vi "Channel Page.vi"(8 "error in (no error)":errorcluster, 11 "Node Ptr":T3 format="%.0x") -> (0 "error out":errorcluster)   [LabVIEW 2011, in "IVI DC Power Supply Custom Device.lvlib"]
uses:
  IVI DC Power Supply Custom Device.lvlib
  <vilib>/NI Veristand/Custom Device API/Custom Device Item Ref.ctl
  current behaviour.ctl
  Global.vi
  <vilib>/NI Veristand/Custom Device Tools/Custom Device Utility Library/NI VeriStand - Search for All Items by GUID.vi
  <vilib>/NI Veristand/Custom Device API/Get Item Property (U16).vi
  <vilib>/NI Veristand/Custom Device API/Get Item Property (Double).vi
  <vilib>/NI Veristand/Custom Device API/Get Item Property (Boolean).vi
  <vilib>/NI Veristand/Custom Device API/Set Item Property (U16).vi
  <vilib>/NI Veristand/Custom Device API/Set Item Property (Double).vi
  <vilib>/NI Veristand/Custom Device Tools/Custom Device Utility Library/NI VeriStand - Search for Item by Name.vi
  <vilib>/NI Veristand/Custom Device API/Set Item Property (Boolean).vi
  <vilib>/NI Veristand/Custom Device API/Custom Device API.lvlib
  <vilib>/NI Veristand/Custom Device Tools/Custom Device Utility Library/Custom Device Utility Library.lvlib
panel:
  in  "Limit Behaviour":T1
  in  "OVP Limt (0.0 Volts)":dbl
  in  "OPV enabled":bool
  in  "Current Limit":dbl
  in  "Output Voltage":dbl
  in  "Channel #":T2(ring)
  in  "Header":cluster{"Section Name":string}={"Section Name"="IVI DC Power Supply Channel Settings"}
  in  "Description":string
  in  "Name":string
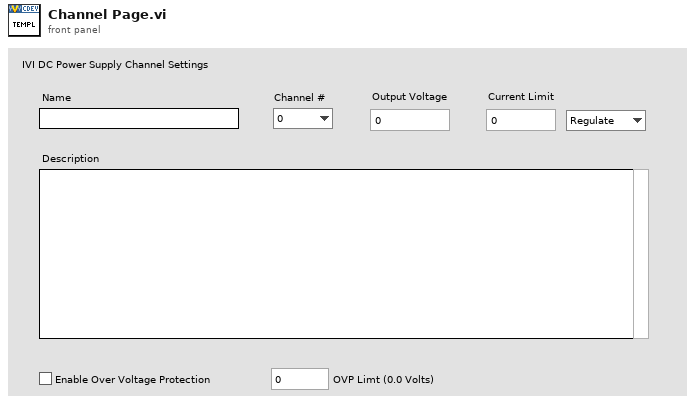
[diagram p1: front panel]
types:
  T1 = typedef "IVI DC Power Supply Custom Device.lvlib/current behaviour.ctl" = enum16{"Regulate", "Trip"}
  T2 = enum16{"0", "1", "2", "3", "4", "5", "6", "7", "8"}
  T3 = typedef "Custom Device API.lvlib/Custom Device Item Ref.ctl" = u64
  T4 = typedef "Custom Device API.lvlib/Custom Device Item Info.ctl" = cluster{"Name":string, "Is Channel":bool, "GUID":string}
  T5 = typedef "Custom Device API.lvlib/Custom Device Commands.ctl" = enum16{"Default", "Item renamed", "Shutdown", "Dynamic button pressed"}
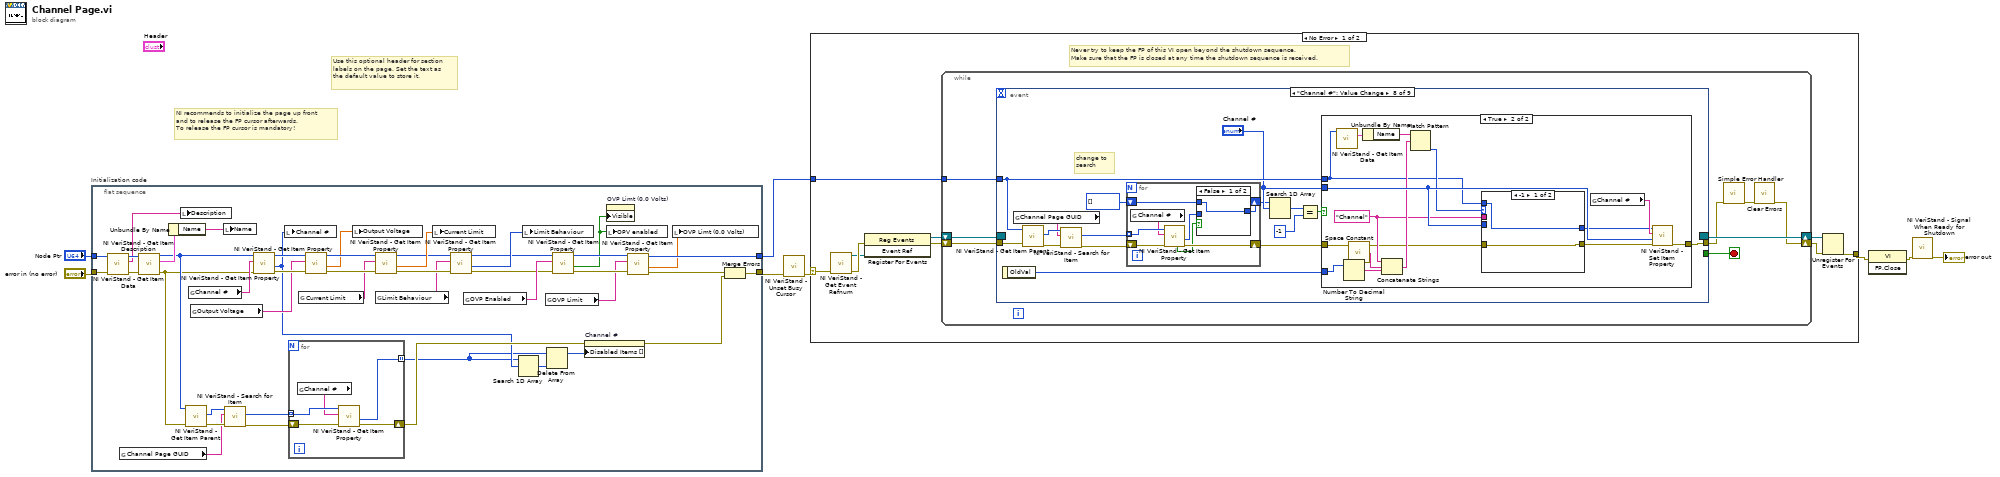
[diagram p0: block diagram]
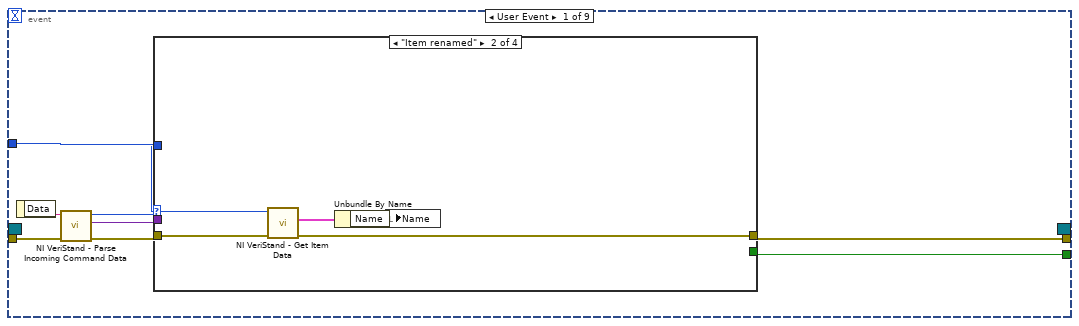
[diagram p2: hidden frame]
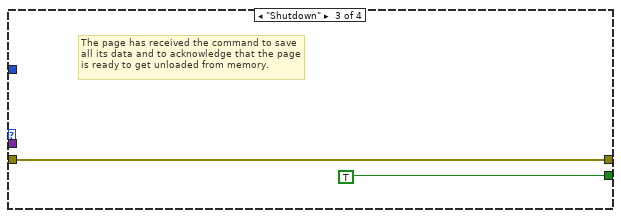
[diagram p4: hidden frame]
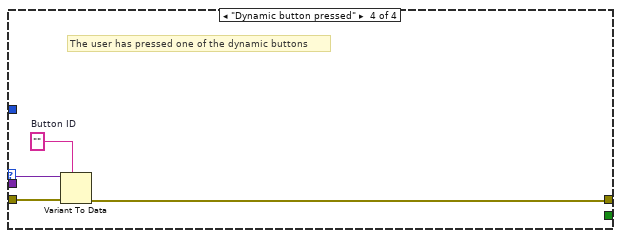
[diagram p5: hidden frame]
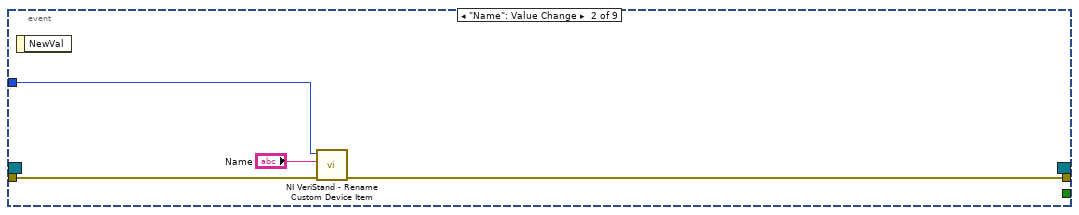
[diagram p6: hidden frame]
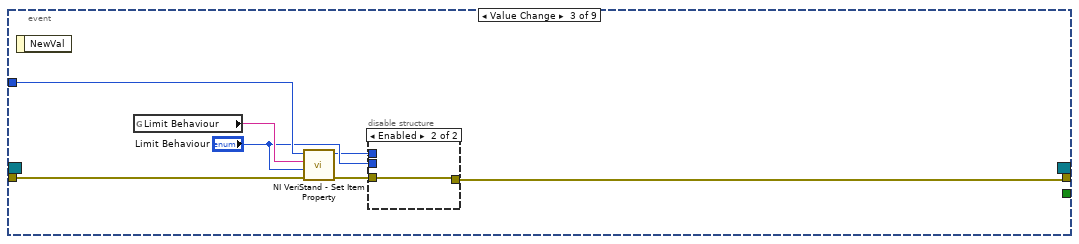
[diagram p7: hidden frame]
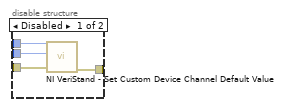
[diagram p8: hidden frame]
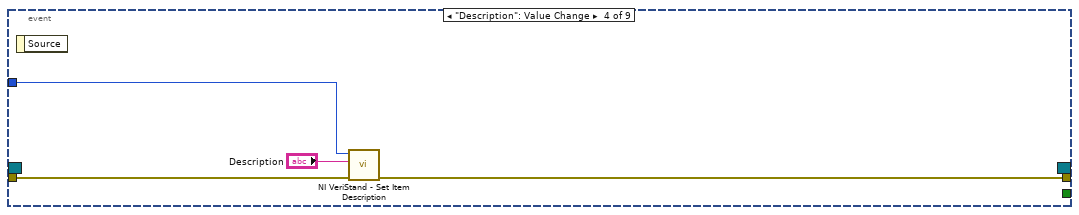
[diagram p9: hidden frame]
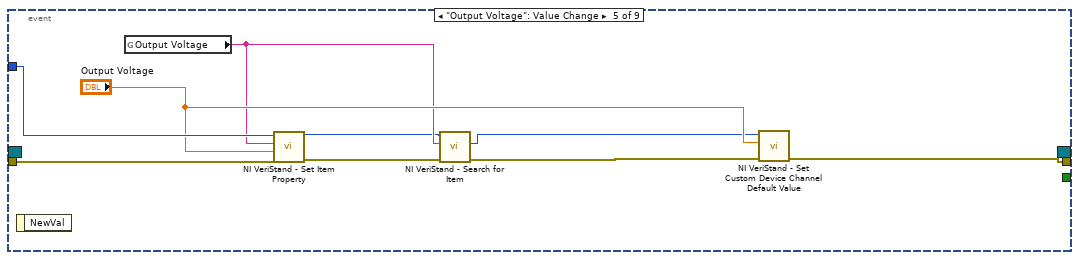
[diagram p10: hidden frame]
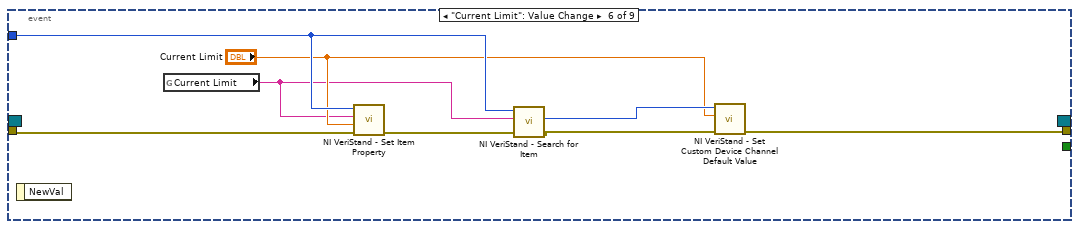
[diagram p11: hidden frame]
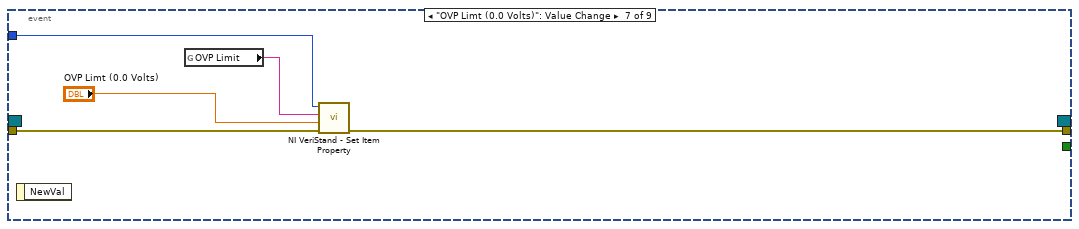
[diagram p12: hidden frame]
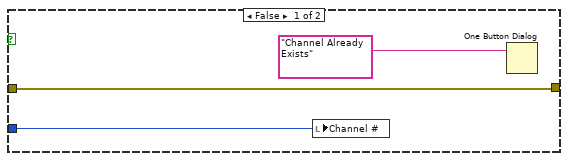
[diagram p13: hidden frame]
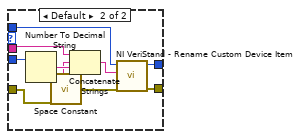
[diagram p14: hidden frame]
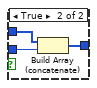
[diagram p15: hidden frame]
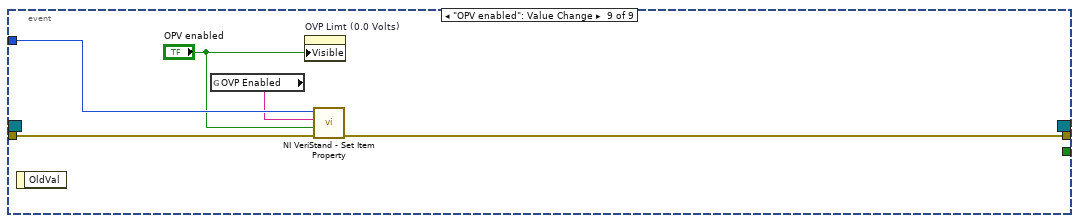
[diagram p16: hidden frame]
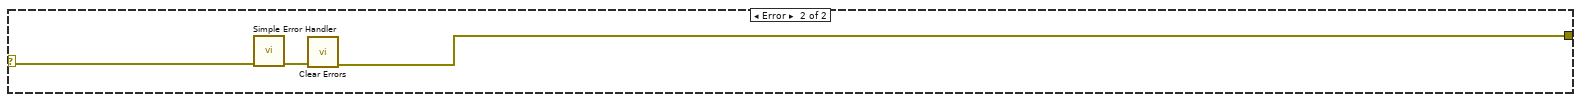
[diagram p17: hidden frame]
diagram:
  # "Use this optional header for section labels on the page. Set the text as the default value to store it."
  # "NI recommends to initialize the page up front\nand to release the FP cursor afterwards.\nTo release the FP cursor is mandatory!"
  n1 = flat-sequence "Initialization code" {
    tunnel: "error in (no error)" -> [w51]
    tunnel: "Node Ptr" -> [w50]
    tunnel: [w34] -> w4
    tunnel: [w24] -> w1
    frame #0 {
      n2 = call <vilib>:"NI VeriStand - Get Item Description.vi"("error in (no error)"=w51, "Item Ref in"=w50) -> ("error out"=w48:errorcluster, "Description"=w49:string, "Item Ref out"=w52:T3)  [unwired: 7 out]
      n3 = global read "Global.vi" "Channel Page GUID"() -> (w9:string)
      n4 = call <vilib>:"NI VeriStand - Get Item Data.vi"("error in (no error)"=w48, "Item Ref in"=w52) -> ("error out"=w35:errorcluster, "Item Info"=w47:T4, "Item Ref out"=w36:T3)  [unwired: 7 out]
      n5 = Unbundle By Name(w47) -> ("Name"=w46:string)
      n6 = local write "Description"(w49) -> ()
      n7 = call <vilib>:"NI VeriStand - Get Item Parent.vi"("error in (no error)"=w35, "Item Ref in"=w36) -> ("error out"=w11:errorcluster, "Parent Ref"=w10:T3)  [unwired: 6 in, 2 out]
      n8 = global read "Global.vi" "Channel #"() -> (w45:string)
      n9 = global read "Global.vi" "Output Voltage"() -> (w42:string)
      n10 = local write "Name"(w46) -> ()
      n11 = call-poly <vilib>:"NI VeriStand - Search for Item.vi"("error in"=w11, "Item GUID"=w9, "Section Ref in"=w10) -> ("error out"=w12:errorcluster, "Item Refs"=w13:T3[])  [unwired: 5 in, 2 out]
      n12 = call-poly <vilib>:"NI VeriStand - Get Item Property.vi"("error in (no error)"=w35, "Property Name"=w45, "Item Ref in"=w36) -> ("error out"=w44:errorcluster, "Value"=w31:u16, "Item Ref out"=w43:T3)  [unwired: 5 in, 1 out]
      n13 = local write "Channel #"(w31) -> ()
      n14 = for {
        tunnel: w13 -> [w57] mode=indexing
        shift-right: [w54] -> w33
        shift-left: w12 -> [w55]
        tunnel: [w53] -> w14 mode=indexing
        n15 = global read "Global.vi" "Channel #"() -> (w56:string)
        n16 = call-poly <vilib>:"NI VeriStand - Get Item Property.vi"("error in (no error)"=w55, "Property Name"=w56, "Item Ref in"=w57) -> ("error out"=w54:errorcluster, "Value"=w53:u16)  [unwired: 5 in, 2 out]
      }
      n17 = global read "Global.vi" "Current Limit"() -> (w39:string)
      n18 = call-poly <vilib>:"NI VeriStand - Get Item Property.vi"("error in (no error)"=w44, "Property Name"=w42, "Item Ref in"=w43) -> ("error out"=w40:errorcluster, "Value"=w38:dbl, "Item Ref out"=w41:T3)  [unwired: 5 in, 1 out]
      n19 = local write "Output Voltage"(w38) -> ()
      n20 = call-poly <vilib>:"NI VeriStand - Get Item Property.vi"("error in (no error)"=w40, "Property Name"=w39, "Item Ref in"=w41) -> ("error out"=w19:errorcluster, "Value"=w37:dbl, "Item Ref out"=w20:T3)  [unwired: 5 in, 1 out]
      n21 = global read "Global.vi" "Limit Behaviour"() -> (w18:string)
      n22 = local write "Current Limit"(w37) -> ()
      n23 = call-poly <vilib>:"NI VeriStand - Get Item Property.vi"("error in (no error)"=w19, "Property Name"=w18, "Item Ref in"=w20) -> ("error out"=w17:errorcluster, "Value"=w16:u16, "Item Ref out"=w15:T3)  [unwired: 5 in, 1 out]
      n24 = global read "Global.vi" "OVP Enabled"() -> (w28:string)
      n25 = Search 1D Array(1D array=w14, element=w31) -> (index of element=w30:i32)  [unwired: 1 in]
      n26 = local write "Limit Behaviour"(w16) -> ()
      n27 = global read "Global.vi" "OVP Limit"() -> (w22:string)
      n28 = Delete From Array(array=w14, index=w30) -> (array with subset deleted=w29:u16[])  [unwired: 1 in, 1 out]
      n29 = call-poly <vilib>:"NI VeriStand - Get Item Property.vi"("error in (no error)"=w17, "Property Name"=w28, "Item Ref in"=w15) -> ("error out"=w26:errorcluster, "Value"=w21:bool, "Item Ref out"=w27:T3)  [unwired: 5 in, 1 out]
      n30 = property on="Channel #" class="Enum (strict)"(error in=w33, "Disabled Items []"=w29) -> (error out=w32:errorcluster)  [unwired: 1 in, 1 out]
      n31 = property on="OVP Limt (0.0 Volts)" class="DigNum (strict)"("Visible"=w21) -> ()  [unwired: 2 in, 2 out]
      n32 = local write "OPV enabled"(w21) -> ()
      n33 = call-poly <vilib>:"NI VeriStand - Get Item Property.vi"("error in (no error)"=w26, "Property Name"=w22, "Item Ref in"=w27) -> ("error out"=w25:errorcluster, "Value"=w23:dbl, "Item Ref out"=w24:T3)  [unwired: 5 in, 1 out]
      n34 = local write "OVP Limt (0.0 Volts)"(w23) -> ()
      n35 = Merge Errors(w25, w32) -> (w34:errorcluster)
    }
  }
  n36 = call <vilib>:"NI VeriStand - Unset Busy Cursor.vi"("error in (no error)"=w4) -> ("error out"=w3:errorcluster)  [unwired: 10 out]
  n37 = case shown="No Error" w3 {
    selector: w3 -> [w58 w201]
    tunnel: [w63 w199] -> w8
    tunnel: w1 -> [w59 _]
    frame No Error {
      # "Never try to keep the FP of this VI open beyond the shutdown sequence.\nMake sure that the FP is closed at any time the shutdown sequence is received."
      n38 = call <vilib>:"NI VeriStand - Get Event Refnum.vi"("error in (no error)"=w58) -> ("error out"=w66:errorcluster, "Event Ref"=w62:refnum<user-event>)  [unwired: 9 out]
      n39 = register-events(error in=w66, w62) -> (reference out=w60:refnum<event-registration>, error out=w61:errorcluster)  [unwired: 1 in]
      n40 = while {
        tunnel: w59 -> [w70]
        shift-right: [w67] -> w64
        shift-left: w61 -> [w73]
        shift-right: [w74] -> w65
        shift-left: w60 -> [w72]
        stop <- w71 stop-if-true
        n41 = event shown="[7] \"Channel #\": Value Change" {
          selector: w72 -> [_ _ _ _ _ _ _ _ _]
          dyn-events: [_ _ _ _ _ _ _ _ _] -> w74
          timeout: _ -> [_ _ _ _ _ _ _ _ _]
          tunnel: w73 -> [w82 w98 w105 w113 w123 w125 w136 w152 w198]
          tunnel: [w78 _ _ _ _ _ _ _ _] -> w71
          tunnel: [w77 w97 w99 w112 w120 w131 w135 w148 w194] -> w69
          tunnel: w70 -> [w76 w96 w104 w114 w122 w128 w133 w146 w197]
          event User Event {
            n42 = event-data() -> ("Data"=w81:string)  [unwired: 1 out]
            n43 = call <vilib>:"NI VeriStand - Parse Incoming Command Data.vi"("error in (no error)"=w82, "Incoming data"=w81) -> ("error out"=w80:errorcluster, "Outgoing data"=w75:variant, "Action"=w79:T5)  [unwired: 7 out]
            n44 = case shown="\"Item renamed\"" w79 {
              tunnel: w80 -> [w83 w88 w89 w94]
              tunnel: [_ _ TRUE _] -> w78
              tunnel: [w83 w85 w89 w91] -> w77
              tunnel: w76 -> [_ w87 _ _]
              tunnel: w75 -> [_ _ _ w93]
              frame "Default", Default {
              }
              frame "Item renamed" {
                n45 = call <vilib>:"NI VeriStand - Get Item Data.vi"("error in (no error)"=w88, "Item Ref in"=w87) -> ("error out"=w85:errorcluster, "Item Info"=w86:T4)  [unwired: 8 out]
                n46 = Unbundle By Name(w86) -> ("Name"=w84:string)
                n47 = local write "Name"(w84) -> ()
              }
              frame "Shutdown" {
                # "The page has received the command to save all its data and to acknowledge that the page is ready to get unloaded from memory."
              }
              frame "Dynamic button pressed" {
                w92 = ""  # Button ID
                # "The user has pressed one of the dynamic buttons"
                n48 = Variant To Data(error in=w94, type=w92, Variant=w93) -> (error out=w91:errorcluster)  [unwired: 1 out]
              }
            }
          }
          event "Name": Value Change {
            n49 = event-data() -> ()  [unwired: 2 out]
            n50 = call <vilib>:"NI VeriStand - Rename Custom Device Item.vi"("error in (no error)"=w98, "New Name"="Name", "Item Ref in"=w96) -> ("error out"=w97:errorcluster)  [unwired: 8 out]
          }
          event Value Change {
            n51 = event-data() -> ()  [unwired: 2 out]
            n52 = global read "Global.vi" "Limit Behaviour"() -> (w103:string)
            n53 = call-poly <vilib>:"NI VeriStand - Set Item Property.vi"("error in (no error)"=w105, "Value"="Limit Behaviour", "Property Name"=w103, "Item Ref in"=w104) -> ("error out"=w102:errorcluster, "Item Ref out"=w100:T3)  [unwired: 5 in, 1 out]
            n54 = disable-structure shown="Enabled" {
              disable-tunnel: w102 -> [w109 w110]
              disable-tunnel: "Limit Behaviour" -> [w108 _]
              disable-tunnel: w100 -> [w107 _]
              disable-tunnel: [w106 w110] -> w99
              frame Disabled {
                n55 = call <vilib>:"NI VeriStand - Set Custom Device Channel Default Value.vi"("error in (no error)"=w109, "Default Value"=w108, "Channel Ref in"=w107) -> ("error out"=w106:errorcluster)  [unwired: 7 in, 1 out]
              }
              frame Enabled {
              }
            }
          }
          event "Description": Value Change {
            n56 = event-data() -> ()  [unwired: 2 out]
            n57 = call <vilib>:"NI VeriStand - Set Item Description.vi"("error in (no error)"=w113, "Description"="Description", "Item Ref in"=w114) -> ("error out"=w112:errorcluster)  [unwired: 8 out]
          }
          event "Output Voltage": Value Change {
            n58 = event-data() -> ()  [unwired: 2 out]
            n59 = global read "Global.vi" "Output Voltage"() -> (w117:string)
            n60 = call-poly <vilib>:"NI VeriStand - Set Item Property.vi"("error in (no error)"=w123, "Value"="Output Voltage", "Property Name"=w117, "Item Ref in"=w122) -> ("error out"=w119:errorcluster, "Item Ref out"=w116:T3)  [unwired: 5 in, 1 out]
            n61 = call-poly <vilib>:"NI VeriStand - Search for Item.vi"("error in"=w119, "Item Name"=w117, "Section Ref in"=w116) -> ("error out"=w118:errorcluster, "Item Ref"=w115:T3)  [unwired: 5 in, 2 out]
            n62 = call <vilib>:"NI VeriStand - Set Custom Device Channel Default Value.vi"("error in (no error)"=w118, "Default Value"="Output Voltage", "Channel Ref in"=w115) -> ("error out"=w120:errorcluster)  [unwired: 7 in, 1 out]
          }
          event "Current Limit": Value Change {
            n63 = event-data() -> ()  [unwired: 2 out]
            n64 = global read "Global.vi" "Current Limit"() -> (w124:string)
            n65 = call-poly <vilib>:"NI VeriStand - Set Item Property.vi"("error in (no error)"=w125, "Value"="Current Limit", "Property Name"=w124, "Item Ref in"=w128) -> ("error out"=w126:errorcluster)  [unwired: 5 in, 2 out]
            n66 = call-poly <vilib>:"NI VeriStand - Search for Item.vi"("error in"=w126, "Item Name"=w124, "Section Ref in"=w128) -> ("error out"=w130:errorcluster, "Item Ref"=w129:T3)  [unwired: 5 in, 2 out]
            n67 = call <vilib>:"NI VeriStand - Set Custom Device Channel Default Value.vi"("error in (no error)"=w130, "Default Value"="Current Limit", "Channel Ref in"=w129) -> ("error out"=w131:errorcluster)  [unwired: 7 in, 1 out]
          }
          event "OVP Limt (0.0 Volts)": Value Change {
            n68 = event-data() -> ()  [unwired: 2 out]
            n69 = global read "Global.vi" "OVP Limit"() -> (w134:string)
            n70 = call-poly <vilib>:"NI VeriStand - Set Item Property.vi"("error in (no error)"=w136, "Value"="OVP Limt (0.0 Volts)", "Property Name"=w134, "Item Ref in"=w133) -> ("error out"=w135:errorcluster)  [unwired: 5 in, 2 out]
          }
          event "Channel #": Value Change {
            # "change to \nsearch"
            n71 = event-data() -> ("OldVal"=w145:T2)  [unwired: 1 out]
            n72 = global read "Global.vi" "Channel Page GUID"() -> (w139:string)
            n73 = call <vilib>:"NI VeriStand - Get Item Parent.vi"("error in (no error)"=w152, "Item Ref in"=w146) -> ("error out"=w138:errorcluster, "Parent Ref"=w140:T3)  [unwired: 6 in, 2 out]
            n74 = call-poly <vilib>:"NI VeriStand - Search for Item.vi"("error in"=w138, "Item GUID"=w139, "Section Ref in"=w140) -> ("error out"=w137:errorcluster, "Item Refs"=w141:T3[])  [unwired: 5 in, 2 out]
            n75 = for {
              tunnel: w141 -> [w189] mode=indexing
              shift-right: [w186] -> w147
              shift-left: w137 -> [w187]
              shift-right: [w185] -> w143
              shift-left: u16[] [] -> [w182]
              n76 = global read "Global.vi" "Channel #"() -> (w188:string)
              n77 = call-poly <vilib>:"NI VeriStand - Get Item Property.vi"("error in (no error)"=w187, "Property Name"=w188, "Item Ref in"=w189) -> ("error out"=w186:errorcluster, "Value"=w183:u16, "Found?"=w184:bool)  [unwired: 5 in, 1 out]
              n78 = case shown="False" w184 {
                tunnel: [w190 w193] -> w185
                tunnel: w183 -> [_ w192]
                tunnel: w182 -> [w190 w191]
                frame False {
                }
                frame True {
                  n79 = Build Array (concatenate)(w191, w192) -> (w193:u16[])
                }
              }
            }
            n80 = Search 1D Array(1D array=w143, element="Channel #") -> (index of element=w151:i32)  [unwired: 1 in]
            n81 = Equal?(x=w151, y=-1) -> (x = y?=w149:bool)
            n82 = case shown="True" w149 {
              tunnel: [w154 w168] -> w148
              tunnel: w147 -> [w154 w156]
              tunnel: w146 -> [_ w159]
              tunnel: "Channel #" -> [_ w169]
              tunnel: w145 -> [w155 w166]
              frame False {
                n83 = local write "Channel #"(w155) -> ()
                n84 = One Button Dialog(message="Channel Already Exists") -> ()  [unwired: 1 in, 1 out]
              }
              frame True {
                w160 = "Channel" ("regular expression")
                n85 = call <vilib>:"NI VeriStand - Get Item Data.vi"("Item Ref in"=w159) -> ("Item Info"=w167:T4)  [unwired: 1 in, 9 out]
                n86 = Number To Decimal String(number=w166) -> (decimal integer string=w164:string)  [unwired: 1 in]
                n87 = call <vilib>:"Space Constant.vi"() -> ("String"=w165:string)
                n88 = Unbundle By Name(w167) -> ("Name"=w163:string)
                n89 = Concatenate Strings(w160, w165, w164) -> (w162:string)
                n90 = Match Pattern(string=w163, regular expression=w162) -> (offset past match=w161:i32)  [unwired: 1 in, 3 out]
                n91 = case shown="-1" w161 {
                  tunnel: w169 -> [_ w180]
                  tunnel: w160 -> [_ w179]
                  tunnel: w159 -> [w172 w177]
                  tunnel: [w172 w176] -> w158
                  tunnel: [w171 w175] -> w157
                  tunnel: w156 -> [w171 w173]
                  frame -1 {
                  }
                  frame Default {
                    n92 = Number To Decimal String(number=w180) -> (decimal integer string=w181:string)  [unwired: 1 in]
                    n93 = call <vilib>:"Space Constant.vi"() -> ("String"=w178:string)
                    n94 = Concatenate Strings(w179, w178, w181) -> (w174:string)
                    n95 = call <vilib>:"NI VeriStand - Rename Custom Device Item.vi"("error in (no error)"=w173, "New Name"=w174, "Item Ref in"=w177) -> ("error out"=w175:errorcluster, "Item Ref out"=w176:T3)  [unwired: 6 in, 1 out]
                  }
                }
                n96 = global read "Global.vi" "Channel #"() -> (w170:string)
                n97 = call-poly <vilib>:"NI VeriStand - Set Item Property.vi"("error in (no error)"=w157, "Value"=w169, "Property Name"=w170, "Item Ref in"=w158) -> ("error out"=w168:errorcluster)  [unwired: 5 in, 2 out]
              }
            }
          }
          event "OPV enabled": Value Change {
            n98 = event-data() -> ()  [unwired: 2 out]
            n99 = global read "Global.vi" "OVP Enabled"() -> (w195:string)
            n100 = property on="OVP Limt (0.0 Volts)" class="DigNum (strict)"("Visible"="OPV enabled") -> ()  [unwired: 2 in, 2 out]
            n101 = call-poly <vilib>:"NI VeriStand - Set Item Property.vi"("error in (no error)"=w198, "Value"="OPV enabled", "Property Name"=w195, "Item Ref in"=w197) -> ("error out"=w194:errorcluster)  [unwired: 5 in, 2 out]
          }
        }
        n102 = call <vilib>:"Simple Error Handler.vi"("error in (no error)"=w69) -> ("error out"=w68:errorcluster)  [unwired: 1 in, 7 out]
        n103 = call <vilib>:"Clear Errors.vi"("error in (no error)"=w68) -> ("error out"=w67:errorcluster)  [unwired: 6 out]
      }
      n104 = Unregister For Events(event registration refnum=w65, error in=w64) -> (error out=w63:errorcluster)
    }
    frame Error {
      n105 = call <vilib>:"Simple Error Handler.vi"("error in (no error)"=w201) -> ("error out"=w200:errorcluster)  [unwired: 1 in, 7 out]
      n106 = call <vilib>:"Clear Errors.vi"("error in (no error)"=w200) -> ("error out"=w199:errorcluster)  [unwired: 6 out]
    }
  }
  n107 = invoke class="VI" method="FP.Close"(error in=w8) -> (error out=w7:errorcluster)  [unwired: 2 in, 2 out]
  n108 = call <vilib>:"NI VeriStand - Signal When Ready for Shutdown.vi"("error in (no error)"=w7) -> ("error out"=→"error out":errorcluster)  [unwired: 10 out]
